vi "Pre Launch Init.vi"(11 "Base Software_Tools in":refnum<class "Base Software.lvclass">) -> (0 "error out":errorcluster, 3 "Base Software_Tools out":refnum<class "Base Software.lvclass">)   [LabVIEW 2019, in "Base Software.lvlib" / "Main.lvlib" / "Base Software.lvclass"]
uses:
  Project/Base Software.lvclass
  builds/Engine/Engine.lvlibp/Project/Engine.lvclass
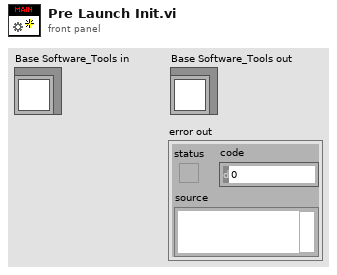
[diagram p1: front panel]
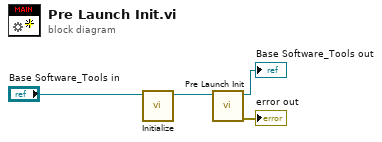
[diagram p0: block diagram]
diagram:
  n1 = call "Initialize.vi"("Base Software in"="Base Software_Tools in") -> ("Base Software out"=w2:refnum<class "Base Software.lvclass">)  [unwired: 9 in, 1 out]
  n2 = call-parent "Pre Launch Init.vi"("Engine_Tools in"=w2) -> ("error out"=→"error out":errorcluster, "Engine_Tools out"=→"Base Software_Tools out":refnum<class "Base Software.lvclass">)  [unwired: 9 in]
